vi "capCalc_calcMean.vi"(6 "signLength":dbl, 7 "signStart":i32, 9 "sigReps":i32, 10 "capCalcCut":i8, 11 "Ch in":dbl[](array[numeric])) -> (3 "capMeanOut":dbl)   [LabVIEW 2021]
uses:
  <vilib>/Analysis/baseanly.llb/Mean (DBL).vi
  <vilib>/Analysis/NI_AALBase.lvlib
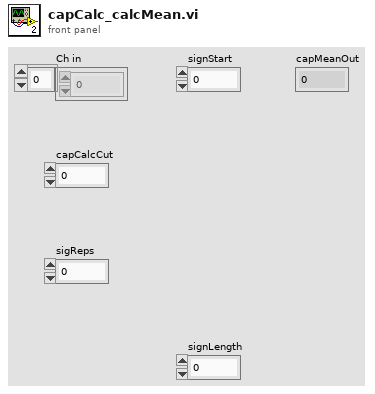
[diagram p1: front panel]
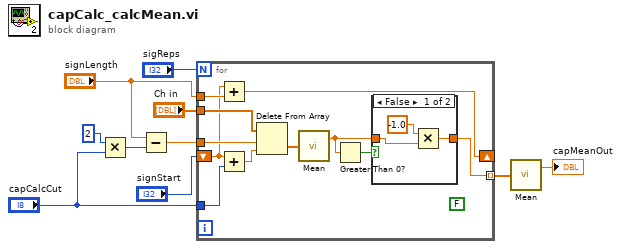
[diagram p0: block diagram]
diagram:
  n1 = Multiply(x=i8 2, y="capCalcCut") -> (x*y=w6:i8)
  n2 = Subtract(x="signLength", y=w6) -> (x-y=w3:dbl)
  n3 = for {
    N: "sigReps" -> [_]
    tunnel: "Ch in" -> [w21]
    tunnel: w3 -> [w19]
    shift-right: [w20] -> _
    shift-left: "signStart" -> [w16]
    tunnel: "signLength" -> [w17]
    tunnel: "capCalcCut" -> [w14]
    tunnel: [w11] -> w8 mode=indexing
    (unwired) FALSE
    n4 = Add(x=w16, y=w17) -> (x+y=w20:dbl)
    n5 = Add(x=w16, y=w14) -> (x+y=w15:dbl)
    n6 = Delete From Array(array=w21, length=w19, index=w15) -> (deleted portion=w18:dbl[])  [unwired: 1 out]
    n7 = call-poly <vilib>:"Mean.vi"("X"=w18) -> ("mean"=w12:dbl)  [unwired: 1 out]
    n8 = Greater Than 0?(x=w12) -> (x > 0?=w13:bool)
    n9 = case shown="False" w13 {
      tunnel: w12 -> [w24 w25]
      tunnel: [w23 w25] -> w11
      frame False {
        n10 = Multiply(x=-1.0, y=w24) -> (x*y=w23:dbl)
      }
      frame True {
      }
    }
  }
  n11 = call-poly <vilib>:"Mean.vi"("X"=w8) -> ("mean"=→"capMeanOut":dbl)  [unwired: 1 out]
